vi "Sample PC Main.vi"(0 "Start":bool, 5 "Pause":bool) -> (4 "Elapsed_Time(s)":dbl, 15 "Error_Out":errorcluster)   [LabVIEW 2021, in "Sample PC Template.lvlib"]
doc: "Sampe CLD Template"
uses:
  Sample PC Template.lvlib
  Typedefs/Queue Operations.ctl
  Typedefs/Timer Details.ctl
  Typedefs/Data Cluster.ctl
  Typedefs/Data.ctl
  Typedefs/User Event Operations.ctl
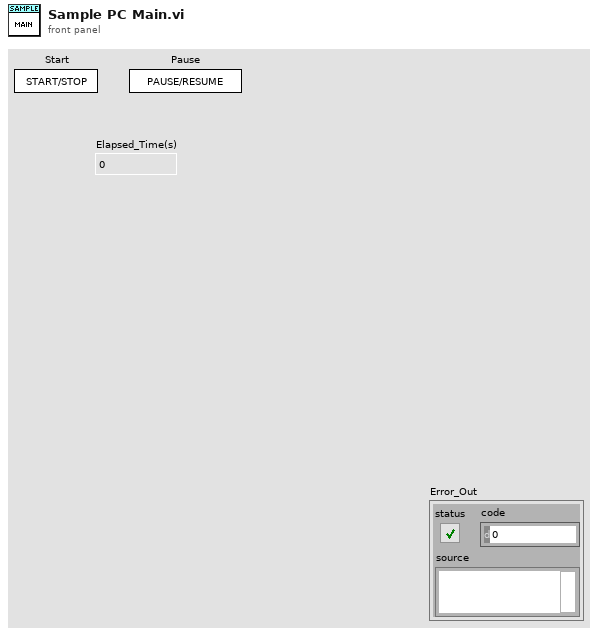
[diagram p1: front panel]
types:
  T1 = typedef "Sample PC Template.lvlib/User Event Operations.ctl" = enum16{"Obtain", "Generate", "Release"}
  T2 = typedef "Sample PC Template.lvlib/Queue Operations.ctl" = enum16{"Create Q", "Enqueue", "Enstack", "Dequeue", "Flush Q", "Release Q"}
  T3 = typedef "Sample PC Template.lvlib/Data.ctl" = cluster{"State":string, "Data":variant}
  T4 = typedef "Sample PC Template.lvlib/Data Cluster.ctl" = cluster{"Timer Details":T5, "Enable Controls ref":refnum<vi>[], "Disable Controls ref":refnum<vi>[], "File Path":path}
  T5 = typedef "Sample PC Template.lvlib/Timer Details.ctl" = cluster{"Elapsed Time":dbl, "Start Time":timestamp, "Started?":bool, "Paused?":bool, "Set Time":dbl, "Previous Time":dbl}
  T6 = enum8{"Enabled", "Disabled", "Disabled and Grayed Out"}
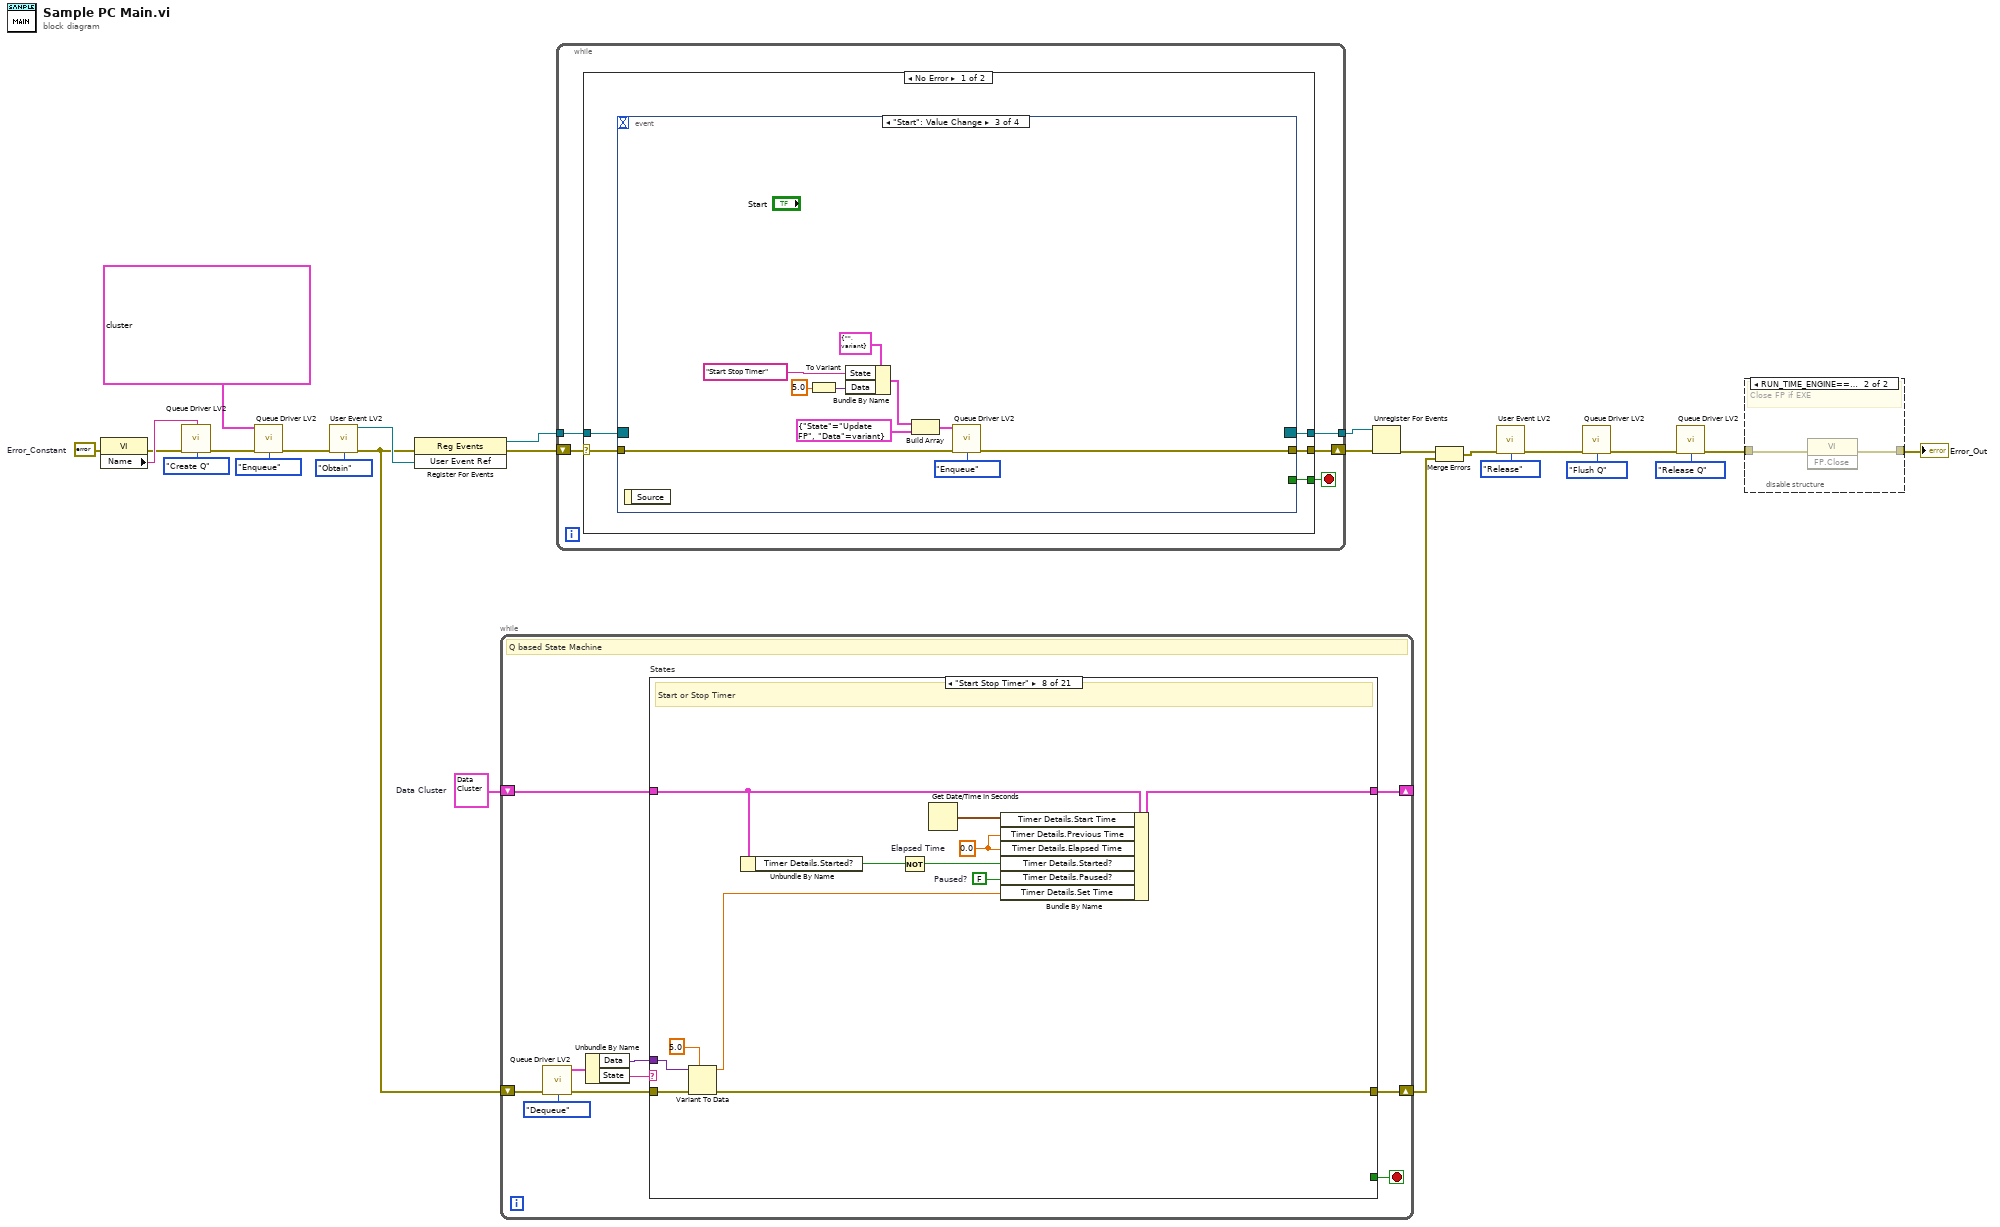
[diagram p0: block diagram]
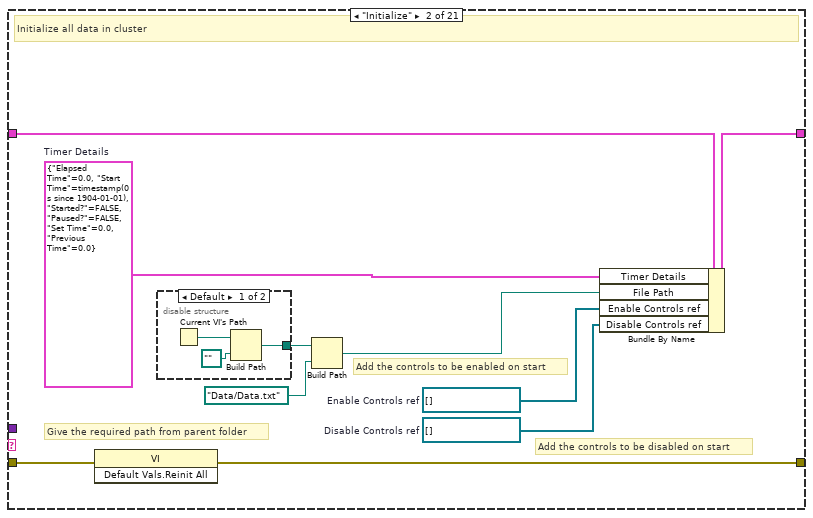
[diagram p3: hidden frame]
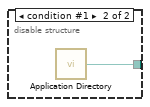
[diagram p4: hidden frame]
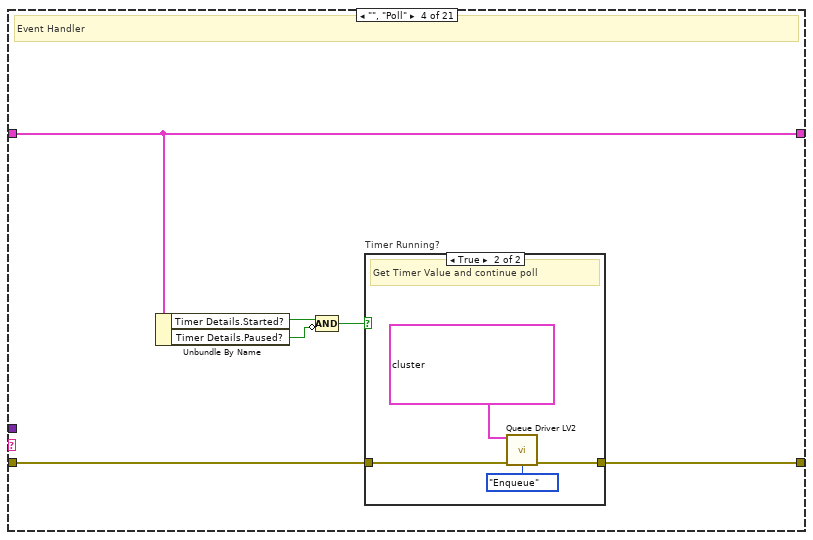
[diagram p6: hidden frame]
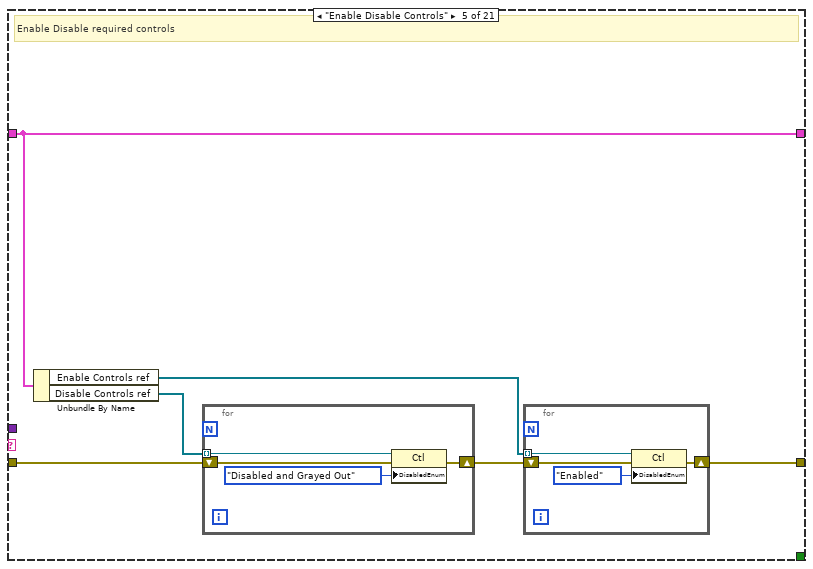
[diagram p8: hidden frame]
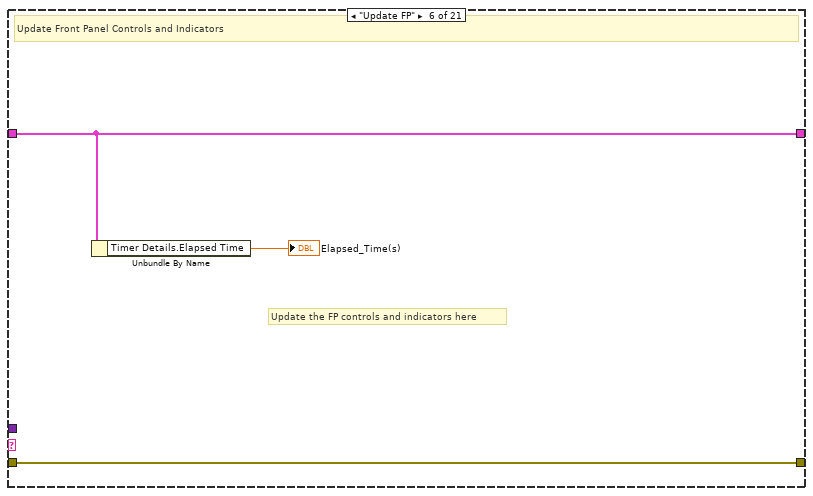
[diagram p9: hidden frame]
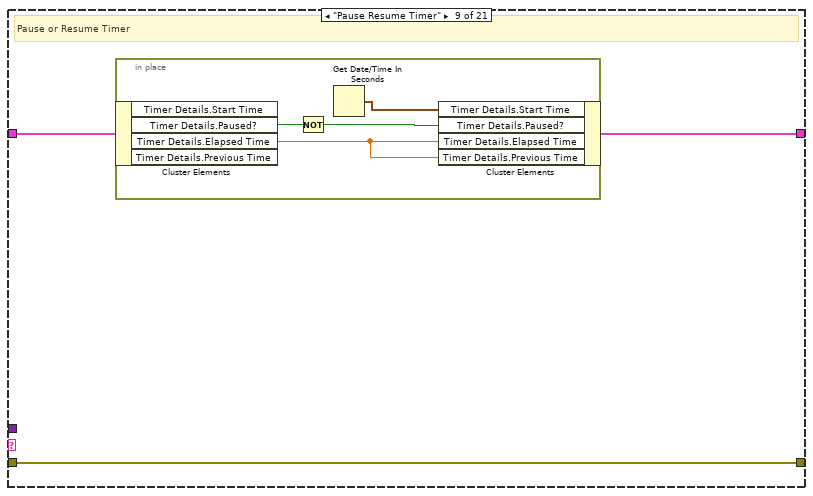
[diagram p11: hidden frame]
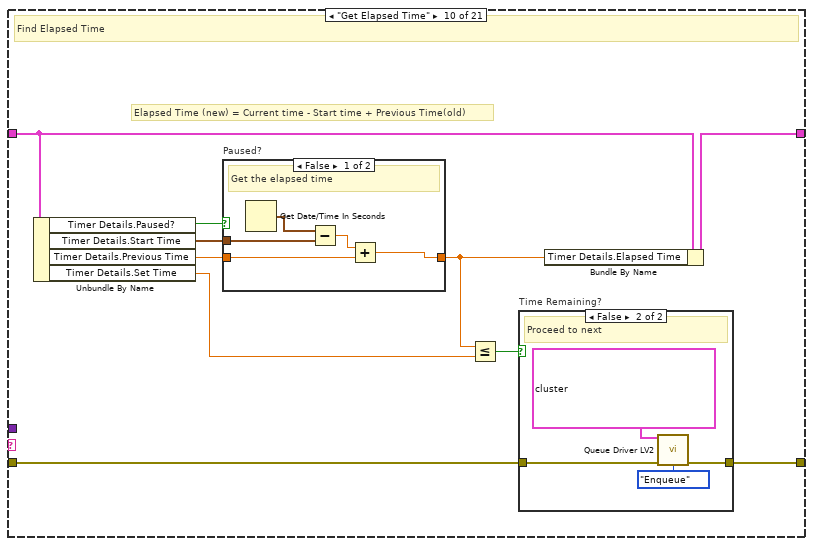
[diagram p12: hidden frame]
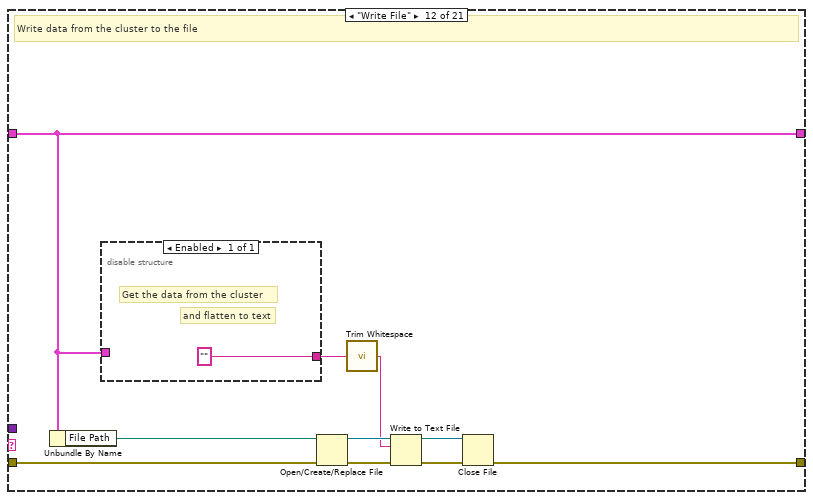
[diagram p16: hidden frame]
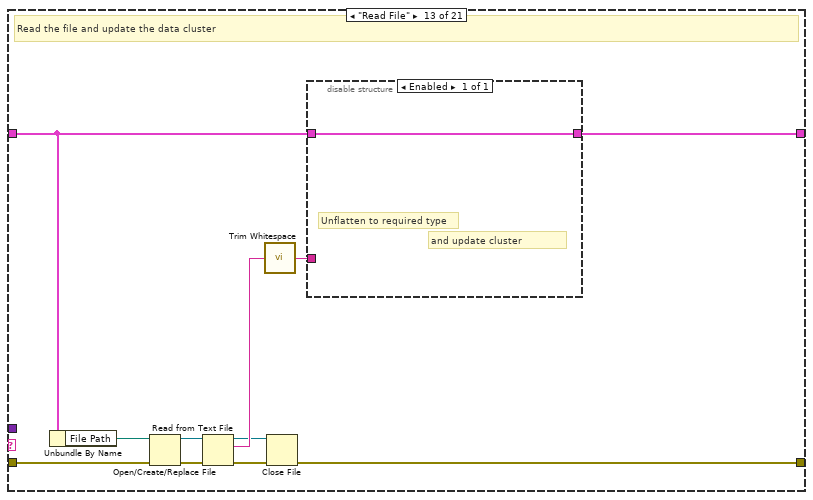
[diagram p17: hidden frame]
diagram:
  w18 = errorcluster {"status"=FALSE, "code"=0, "source"=""}  # Error_Constant
  w20 = T4 {"Timer Details"={"Elapsed Time"=0.0, "Start Time"=timestamp(0 s since 1904-01-01), "Started?"=FALSE, "Paused?"=FALSE, "Set Time"=0.0, "Previous Time"=0.0}, "Enable Controls ref"=[], "Disable Controls ref"=[], "File Path"=path ""}  # Data Cluster
  n1 = property on="Property Node" class="VI"(error in=w18) -> (error out=w24:errorcluster, "Name"=w25:string)  [unwired: 1 in, 1 out]
  n2 = call "Queue Driver LV2.vi"("Name"=w25, "Error In"=w24, "Operation"=Queue_Operations."Create Q") -> ("error out"=w26:errorcluster)  [unwired: 11 in, 1 out]
  n3 = call "Queue Driver LV2.vi"("States"=T3[] [{"State"="Initialize", "Data"=variant}, {"State"="Read File", "Data"=variant}, {"State"="Enable Disable Controls", "Data"=variant}, {"State"="Update FP", "Data"=variant}], "Error In"=w26, "Operation"=Queue_Operations."Enqueue") -> ("error out"=w7:errorcluster)  [unwired: 11 in, 1 out]
  n4 = call "User Event LV2.vi"("Error In"=w7, "Operation"=User_Event_Operations."Obtain") -> ("User Event Ref"=w16:refnum<user-event>, "Error Out"=w8:errorcluster)  [unwired: 12 in]
  n5 = register-events(error in=w8, w16) -> (reference out=w14:refnum<event-registration>, error out=w17:errorcluster)  [unwired: 1 in]
  n6 = while {
    shift-right: [w32] -> w2
    shift-left: w8 -> [w36]
    shift-right: [w30] -> _
    shift-left: w20 -> [w31]
    stop <- w29 stop-if-true
    # "Q based State Machine"
    n7 = call "Queue Driver LV2.vi"("Error In"=w36, "Operation"=Queue_Operations."Dequeue") -> ("Dequeued State"=w33:T3, "error out"=w35:errorcluster)  [unwired: 12 in]
    n8 = Unbundle By Name(w33) -> ("Data"=w27:variant, "State"=w28:string)
    n9 = case "States" shown="\"Start Stop Timer\"" w28 {
      selector: w28 -> [_ _ _ _ _ _ _ _ _ _ _ _ _ _ _ _ _ _ w199 _ _]
      tunnel: w35 -> [w38 w48 w54 w60 w71 w82 w84 w85 w99 w113 w126 w132 w148 w151 w153 w155 w160 w183 w203 w220 w222]
      tunnel: [w38 w39 w54 w59 w67 w82 w84 w86 w99 w105 w126 w130 w140 w151 w153 w155 w157 w180 w200 w220 w223] -> w32
      tunnel: w31 -> [w37 w47 w53 w58 w66 w81 w83 w96 w98 w107 w125 w128 w142 w150 w152 w154 w168 w191 w211 w219 w226]
      tunnel: [w37 w46 w53 w58 w66 w81 w83 w95 w97 w106 w125 w128 w141 w150 w152 w154 w168 w191 w211 w219 w226] -> w30
      tunnel: [_ _ _ _ _ _ _ _ _ _ _ _ _ _ _ _ TRUE TRUE _ _ TRUE] -> w29
      tunnel: w27 -> [_ _ _ _ _ _ _ w88 _ _ _ _ _ _ _ _ _ w179 _ _ _]
      frame "/***Initialize***/" {
      }
      frame "Initialize" {
        w44 = refnum<vi>[] []  # Disable Controls ref
        w45 = refnum<vi>[] []  # Enable Controls ref
        w40 = T5 {"Elapsed Time"=0.0, "Start Time"=timestamp(0 s since 1904-01-01), "Started?"=FALSE, "Paused?"=FALSE, "Set Time"=0.0, "Previous Time"=0.0}  # Timer Details
        # "Give the required path from parent folder"
        # "Add the controls to be enabled on start"
        # "Add the controls to be disabled on start"
        # "Initialize all data in cluster"
        n10 = invoke on="Invoke Node" class="VI" method="Default Vals.Reinit All"(error in=w48) -> (error out=w39:errorcluster)  [unwired: 2 in, 2 out]
        n11 = disable-structure "Conditional Disable Structure" shown="Default" {
          disable-tunnel: [w49 w52] -> w43
          frame condition #0 (active) {
            n12 = Current VI's Path() -> (path=w51:path)
            n13 = Build Path(base path=w51, name or relative path=path "..") -> (appended path=w49:path)
          }
          frame condition #1 {
            n14 = call <vilib>:"Application Directory.vi"() -> ("Application Directory"=w52:path)
          }
        }
        n15 = Build Path(base path=w43, name or relative path=path "Data/Data.txt") -> (appended path=w41:path)
        n16 = Bundle By Name(cluster=w47, "Timer Details"=w40, "File Path"=w41, "Enable Controls ref"=w45, "Disable Controls ref"=w44) -> (w46:T4)
      }
      frame "/***FP Related***/" {
      }
      frame "", "Poll" {
        # "Event Handler"
        n17 = Unbundle By Name(w58) -> ("Timer Details.Started?"=w56:bool, "Timer Details.Paused?"=w57:bool)
        n18 = Compound Arithmetic op=AND(w56, invert w57) -> (w55:bool)
        n19 = case "Timer Running?" shown="True" w55 {
          tunnel: w60 -> [w61 w63]
          tunnel: [w61 w65] -> w59
          frame False {
            # "Timer Not Running, so keep polling"
          }
          frame True {
            # "Get Timer Value and continue poll"
            n20 = call "Queue Driver LV2.vi"("States"=T3[] [{"State"="Get Elapsed Time", "Data"=variant}, {"State"="Update FP", "Data"=variant}], "Error In"=w63, "Operation"=Queue_Operations."Enqueue") -> ("error out"=w65:errorcluster)  [unwired: 11 in, 1 out]
          }
        }
      }
      frame "Enable Disable Controls" {
        # "Enable Disable required controls"
        n21 = Unbundle By Name(w66) -> ("Enable Controls ref"=w68:refnum<vi>[], "Disable Controls ref"=w70:refnum<vi>[])
        n22 = for {
          shift-right: [w78] -> w69
          shift-left: w71 -> [w79]
          tunnel: w70 -> [w77] mode=indexing
          n23 = property on="Property Node" class="Ctl"(reference=w77, error in=w79, "DisabledEnum"=T6."Disabled and Grayed Out" ("Disabled")) -> (error out=w78:errorcluster)  [unwired: 1 out]
        }
        n24 = for {
          shift-right: [w74] -> w67
          shift-left: w69 -> [w75]
          tunnel: w68 -> [w73] mode=indexing
          n25 = property on="Property Node" class="Ctl"(reference=w73, error in=w75, "DisabledEnum"=T6."Enabled" ("Disabled")) -> (error out=w74:errorcluster)  [unwired: 1 out]
        }
      }
      frame "Update FP" {
        # "Update the FP controls and indicators here"
        # "Update Front Panel Controls and Indicators"
        n26 = Unbundle By Name(w81) -> ("Timer Details.Elapsed Time"=→"Elapsed_Time(s)":dbl)
      }
      frame "/***Timer Functions***/" {
      }
      frame "Start Stop Timer" {
        w93 = FALSE  # Paused?
        w90 = 0.0  # Elapsed Time
        # "Start or Stop Timer"
        n27 = Variant To Data(error in=w85, type=5.0 ("Timer Details.Set Time"), Variant=w88) -> (data=w87:dbl, error out=w86:errorcluster)
        n28 = Unbundle By Name(w96) -> ("Timer Details.Started?"=w94:bool)
        n29 = Not(x=w94) -> (.not. x?=w91:bool)
        n30 = Get Date/Time In Seconds() -> (seconds since 1Jan1904=w92:timestamp)
        n31 = Bundle By Name(cluster=w96, "Timer Details.Start Time"=w92, "Timer Details.Previous Time"=w90, "Timer Details.Elapsed Time"=w90, "Timer Details.Started?"=w91, "Timer Details.Paused?"=w93, "Timer Details.Set Time"=w87) -> (w95:T4)
      }
      frame "Pause Resume Timer" {
        # "Pause or Resume Timer"
        n32 = in-place "In Place Element Structure" {
          n33 = in-place-cluster #1(w98) -> ("Timer Details.Paused?"=w103:bool, "Timer Details.Elapsed Time"=w100:dbl)  [unwired: 2 out]
          n34 = Not(x=w103) -> (.not. x?=w102:bool)
          n35 = Get Date/Time In Seconds() -> (seconds since 1Jan1904=w101:timestamp)
          n36 = in-place-cluster #1("Timer Details.Start Time"=w101, "Timer Details.Paused?"=w102, "Timer Details.Elapsed Time"=w100, "Timer Details.Previous Time"=w100) -> (w97:T4)
        }
      }
      frame "Get Elapsed Time" {
        # "Elapsed Time (new) = Current time - Start time + Previous Time(old)"
        # "Find Elapsed Time"
        n37 = Unbundle By Name(w107) -> ("Timer Details.Paused?"=w108:bool, "Timer Details.Start Time"=w112:timestamp, "Timer Details.Previous Time"=w111:dbl, "Timer Details.Set Time"=w109:dbl)
        n38 = case "Paused?" shown="False" w108 {
          tunnel: w112 -> [w123 _]
          tunnel: w111 -> [w121 w124]
          tunnel: [w119 w124] -> w110
          frame False {
            # "Get the elapsed time"
            n39 = Get Date/Time In Seconds() -> (seconds since 1Jan1904=w120:timestamp)
            n40 = Subtract(x=w120, y=w123) -> (x-y=w122:dbl)
            n41 = Add(x=w122, y=w121) -> (x+y=w119:dbl)
          }
          frame True {
            # "Give same value if timer paused"
          }
        }
        n42 = Less Or Equal?(x=w110, y=w109) -> (x <= y?=w104:bool)
        n43 = case "Time Remaining?" shown="False" w104 {
          tunnel: w113 -> [w114 w118]
          tunnel: [w114 w117] -> w105
          frame True {
            # "Continue"
          }
          frame False {
            # "Proceed to next"
            n44 = call "Queue Driver LV2.vi"("States"=T3[] [{"State"="Start Stop Timer", "Data"=variant}, {"State"="Goto Next Step", "Data"=variant}], "Error In"=w118, "Operation"=Queue_Operations."Enqueue") -> ("error out"=w117:errorcluster)  [unwired: 11 in, 1 out]
          }
        }
        n45 = Bundle By Name(cluster=w107, "Timer Details.Elapsed Time"=w110) -> (w106:T4)
      }
      frame "/***File Operations***/" {
      }
      frame "Write File" {
        # "Write data from the cluster to the file"
        n46 = Unbundle By Name(w128) -> ("File Path"=w131:path)
        n47 = disable-structure "Diagram Disable Structure" shown="Enabled" {
          disable-tunnel: [""] -> w129
          disable-tunnel: w128 -> [_]
          frame Enabled {
            # "Get the data from the cluster"
            # "and flatten to text"
          }
        }
        n48 = Open/Create/Replace File(file path (use dialog)=w131, error in=w132) -> (refnum out=w133:refnum<file>, error out=w134:errorcluster)  [unwired: 4 in, 1 out]
        n49 = call <vilib>:"Trim Whitespace.vi"("string"=w129) -> ("trimmed string"=w127:string)  [unwired: 1 in]
        n50 = Write to Text File(file (use dialog)=w133, text=w127, error in=w134) -> (refnum out=w136:refnum<file>, error out=w135:errorcluster)  [unwired: 1 in, 1 out]
        n51 = Close File(refnum=w136, error in=w135) -> (error out=w130:errorcluster)  [unwired: 1 out]
      }
      frame "Read File" {
        # "Read the file and update the data cluster"
        n52 = Unbundle By Name(w142) -> ("File Path"=w144:path)
        n53 = Open/Create/Replace File(file path (use dialog)=w144, error in=w148) -> (refnum out=w145:refnum<file>, error out=w147:errorcluster)  [unwired: 4 in, 1 out]
        n54 = Read from Text File(file (use dialog)=w145, error in=w147) -> (refnum out=w139:refnum<file>, text=w143:string, error out=w146:errorcluster)  [unwired: 2 in, 1 out]
        n55 = call <vilib>:"Trim Whitespace.vi"("string"=w143) -> ("trimmed string"=w138:string)  [unwired: 1 in]
        n56 = Close File(refnum=w139, error in=w146) -> (error out=w140:errorcluster)  [unwired: 1 out]
        n57 = disable-structure "Diagram Disable Structure" shown="Enabled" {
          disable-tunnel: w138 -> [_]
          disable-tunnel: [w149] -> w141
          disable-tunnel: w142 -> [w149]
          frame Enabled {
            # "Unflatten to required type"
            # "and update cluster"
          }
        }
      }
      frame "/***Functionality***/" {
      }
      frame "Goto Next Step" {
        # "Handle what to do next after time elapsed"
        # "Next step after timer elapsed"
      }
      frame "/***Error***/" {
      }
      frame "Error" {
        # "Handle Errors"
        n58 = Unbundle By Name(w160) -> ("code"=w156:i32, "source"=w164:string)
        n59 = call <vilib>:"Clear Errors.vi"("error in (no error)"=w160, "specific error code to clear (0: all)"=w156) -> ("error out"=w166:errorcluster)  [unwired: 4 in, 1 out]
        n60 = Format Into String(format string="Error occurred!\nError Code: %d\nError Source: %s\n\nDo you wish to continue?", error in=w166, w156, w164) -> (resulting string=w163:string, error out=w158:errorcluster)  [unwired: 1 in]
        n61 = Two Button Dialog(message=w163, 1:"Exit" ("F button name (\"Cancel\")"), 2:"Continue" ("T button name (\"OK\")")) -> (T button?=w159:bool)
        n62 = case "Continue?" shown="False" w159 {
          tunnel: w158 -> [w173 w175]
          tunnel: [w170 w175] -> w157
          frame False {
            # "Exit"
            n63 = call "Queue Driver LV2.vi"("Error In"=w173, "Operation"=Queue_Operations."Flush Q") -> ("error out"=w171:errorcluster)  [unwired: 12 in, 1 out]
            n64 = call "Queue Driver LV2.vi"("States"=T3[] [{"State"="Write File", "Data"=variant}, {"State"="Initialize", "Data"=variant}, {"State"="Enable Disable Controls", "Data"=variant}, {"State"="Update FP", "Data"=variant}, {"State"="Exit", "Data"=variant}], "Error In"=w171, "Operation"=Queue_Operations."Enqueue") -> ("error out"=w170:errorcluster)  [unwired: 11 in, 1 out]
          }
          frame True {
            # "Continue"
          }
        }
      }
      frame "Producer Error" {
        # "Handle Errors"
        n65 = Variant To Data(error in=w183, type=errorcluster {"status"=FALSE, "code"=0, "source"=""} ("error out"), Variant=w179) -> (data=w177:errorcluster, error out=w189:errorcluster)
        n66 = Unbundle By Name(w177) -> ("code"=w178:i32, "source"=w187:string)
        n67 = Format Into String(format string="Error occurred!\nError Code: %d\nError Source: %s\n\nDo you wish to continue?", error in=w189, w178, w187) -> (resulting string=w186:string, error out=w181:errorcluster)  [unwired: 1 in]
        n68 = Two Button Dialog(message=w186, 1:"Exit" ("F button name (\"Cancel\")"), 2:"Continue" ("T button name (\"OK\")")) -> (T button?=w182:bool)
        n69 = case "Continue?" shown="False" w182 {
          tunnel: w181 -> [w196 w198]
          tunnel: [w193 w198] -> w180
          frame False {
            # "Exit"
            n70 = call "Queue Driver LV2.vi"("Error In"=w196, "Operation"=Queue_Operations."Flush Q") -> ("error out"=w194:errorcluster)  [unwired: 12 in, 1 out]
            n71 = call "Queue Driver LV2.vi"("States"=T3[] [{"State"="Write File", "Data"=variant}, {"State"="Initialize", "Data"=variant}, {"State"="Enable Disable Controls", "Data"=variant}, {"State"="Update FP", "Data"=variant}, {"State"="Exit", "Data"=variant}], "Error In"=w194, "Operation"=Queue_Operations."Enqueue") -> ("error out"=w193:errorcluster)  [unwired: 11 in, 1 out]
          }
          frame True {
            # "Continue"
          }
        }
      }
      frame "Developer Error", Default {
        # "You can remove this case after development, and make \"Poll\" as Default case"
        # "Handle Errors"
        n72 = Unbundle By Name(w203) -> ("code"=w208:i32, "source"=w207:string)
        n73 = call <vilib>:"Clear Errors.vi"("error in (no error)"=w203, "specific error code to clear (0: all)"=w208) -> ("error out"=w210:errorcluster)  [unwired: 4 in, 1 out]
        n74 = Format Into String(format string="DEVELOPER ERROR\nState \"%s\" not found!!\nError Code: %d\nError Source: %s\n\nDo you wish to continue?", error in=w210, w199, w208, w207) -> (resulting string=w206:string, error out=w201:errorcluster)  [unwired: 1 in]
        n75 = Two Button Dialog(message=w206, 1:"Exit" ("F button name (\"Cancel\")"), 2:"Continue" ("T button name (\"OK\")")) -> (T button?=w202:bool)
        n76 = case "Continue?" shown="False" w202 {
          tunnel: w201 -> [w216 w218]
          tunnel: [w213 w218] -> w200
          frame False {
            # "Exit"
            n77 = call "Queue Driver LV2.vi"("Error In"=w216, "Operation"=Queue_Operations."Flush Q") -> ("error out"=w214:errorcluster)  [unwired: 12 in, 1 out]
            n78 = call "Queue Driver LV2.vi"("States"=T3[] [{"State"="Exit", "Data"=variant}], "Error In"=w214, "Operation"=Queue_Operations."Enqueue") -> ("error out"=w213:errorcluster)  [unwired: 11 in, 1 out]
          }
          frame True {
            # "Continue"
          }
        }
      }
      frame "/***Exit***/" {
      }
      frame "Exit" {
        # "Exit the State Machine"
        n79 = call "User Event LV2.vi"("Data"=T3 {"State"="Exit", "Data"=variant}, "Error In"=w222, "Operation"=User_Event_Operations."Generate") -> ("Error Out"=w223:errorcluster)  [unwired: 11 in, 1 out]
      }
    }
  }
  n80 = while {
    shift-right: [w230] -> w10
    shift-left: w17 -> [w231]
    tunnel: w14 -> [w229]
    tunnel: [w227] -> w9
    stop <- w228 stop-if-true
    n81 = case shown="No Error" w231 {
      selector: w231 -> [w236 w266]
      tunnel: [w235 w269] -> w230
      tunnel: w229 -> [w234 _]
      tunnel: [w233 FALSE] -> w228
      tunnel: [w232 _] -> w227
      frame No Error {
        n82 = event shown="[2] \"Start\": Value Change" {
          selector: w234 -> [_ _ _ _]
          dyn-events: [_ _ _ _] -> w232
          timeout: _ -> [_ _ _ _]
          tunnel: w236 -> [w239 w243 w253 w258]
          tunnel: [w240 w244 w254 w257] -> w235
          tunnel: [_ _ _ w256] -> w233
          event Panel Close? {
            n83 = event-data() -> ()  [unwired: 1 in, 4 out]
            n84 = call "Queue Driver LV2.vi"("States"=T3[] [{"State"="Write File", "Data"=variant}, {"State"="Exit", "Data"=variant}], "Error In"=w239, "Operation"=Queue_Operations."Enqueue") -> ("error out"=w240:errorcluster)  [unwired: 11 in, 1 out]
            n85 = event-data ("Event Filter Node")("Discard?"=TRUE) -> ()  [unwired: 1 in, 1 out]
          }
          event "Pause": Value Change {
            n86 = event-data() -> ()  [unwired: 1 in, 1 out]
            n87 = call "Queue Driver LV2.vi"("States"=T3[] [{"State"="Pause Resume Timer", "Data"=variant}, {"State"="Update FP", "Data"=variant}], "Error In"=w243, "Operation"=Queue_Operations."Enqueue") -> ("error out"=w244:errorcluster)  [unwired: 11 in, 1 out]
          }
          event "Start": Value Change {
            n88 = event-data() -> ()  [unwired: 1 in, 1 out]
            n89 = To Variant(anything=5.0 ("Timer Details.Set Time")) -> (Variant=w250:variant)
            n90 = Bundle By Name(cluster=T3 {"State"="", "Data"=variant} ("Cluster"), "State"="Start Stop Timer", "Data"=w250) -> (w248:T3)
            n91 = Build Array(w248, T3 {"State"="Update FP", "Data"=variant} ("Cluster")) -> (w247:T3[])
            n92 = call "Queue Driver LV2.vi"("States"=w247, "Error In"=w253, "Operation"=Queue_Operations."Enqueue") -> ("error out"=w254:errorcluster)  [unwired: 11 in, 1 out]
          }
          event User Event {
            n93 = event-data() -> ("State"=w260:string, "Data"=w259:variant)  [unwired: 1 in]
            n94 = case shown="\"Exit\"" w260 {
              tunnel: w259 -> [_ _]
              tunnel: [w262 w264] -> w257
              tunnel: w258 -> [w262 w264]
              tunnel: [FALSE TRUE] -> w256
              frame Default {
              }
              frame "Exit" {
              }
            }
          }
        }
      }
      frame Error {
        n95 = To Variant(anything=w266) -> (Variant=w267:variant)
        n96 = Unbundle By Name(w266) -> ("code"=w265:i32)
        n97 = Bundle By Name(cluster=T3 {"State"="", "Data"=variant} ("Cluster"), "State"="Producer Error", "Data"=w267) -> (w274:T3)
        n98 = call <vilib>:"Clear Errors.vi"("error in (no error)"=w266, "specific error code to clear (0: all)"=w265) -> ("error out"=w268:errorcluster)  [unwired: 4 in, 1 out]
        n99 = Build Array(w274) -> (w273:T3[])
        n100 = call "Queue Driver LV2.vi"("States"=w273, "Error In"=w268, "Operation"=Queue_Operations."Enqueue") -> ("error out"=w269:errorcluster)  [unwired: 11 in, 1 out]
      }
    }
  }
  n101 = Unregister For Events(event registration refnum=w9, error in=w10) -> (error out=w4:errorcluster)
  n102 = Merge Errors(w4, w2) -> (w3:errorcluster)
  n103 = call "User Event LV2.vi"("Error In"=w3, "Operation"=User_Event_Operations."Release") -> ("Error Out"=w5:errorcluster)  [unwired: 12 in, 1 out]
  n104 = call "Queue Driver LV2.vi"("Error In"=w5, "Operation"=Queue_Operations."Flush Q") -> ("error out"=w11:errorcluster)  [unwired: 12 in, 1 out]
  n105 = call "Queue Driver LV2.vi"("Error In"=w11, "Operation"=Queue_Operations."Release Q") -> ("error out"=w1:errorcluster)  [unwired: 12 in, 1 out]
  n106 = disable-structure "Conditional Disable Structure" shown="RUN_TIME_ENGINE==True" {
    disable-tunnel: w1 -> [w276 w278]
    disable-tunnel: [w276 w277] -> w19
    frame condition #0 (active) {
    }
    frame condition #1 {
      # "Close FP if EXE"
      n107 = invoke on="Invoke Node" class="VI" method="FP.Close"(error in=w278) -> (error out=w277:errorcluster)  [unwired: 2 in, 2 out]
    }
  }
  "Error_Out" <- w19
